vi "Midi Select Patch.vi"(5 "Patch?":i32, 6 "Channel":i32, 7 "MIDI out handle":i32) -> (0 "Win32 error code":i32, 3 "Duplicate MIDI handle":i32)   [LabVIEW 2016]
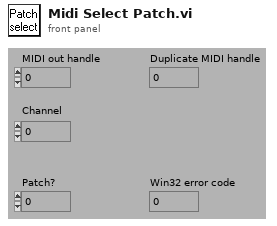
[diagram p1: front panel]
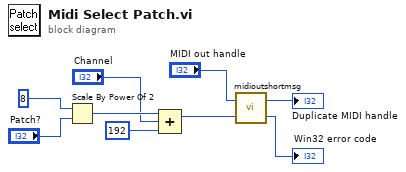
[diagram p0: block diagram]
diagram:
  n1 = Scale By Power Of 2(n=8, x="Patch?") -> (x*2^n=w9:i32)
  n2 = Compound Arithmetic op=ADD(w9, "Channel", 192 ("data")) -> (w4:i32)
  n3 = call "midioutshortmsg.vi"("Data"=w4, "MIDI output handle"="MIDI out handle") -> ("Win32 error code"=→"Win32 error code":i32, "Duplicate MIDI output handle"=→"Duplicate MIDI handle":i32)
